vi "Create Rubix Cube in 3D Pic Control.vi"(8 "error in (no error)":errorcluster, 10 "Rubix Array":string[][](array[string])) -> (0 "error out":errorcluster, 2 "Rubix Array":refnum<vi>[][](array[refnum]), 3 "Scene:New Object":refnum<vi>)   [LabVIEW 2019]
uses:
  <vilib>/picture/3D Picture Control/Object/Create Object (name).vi
  <vilib>/picture/3D Picture Control/NI_3D Picture Control.lvlib
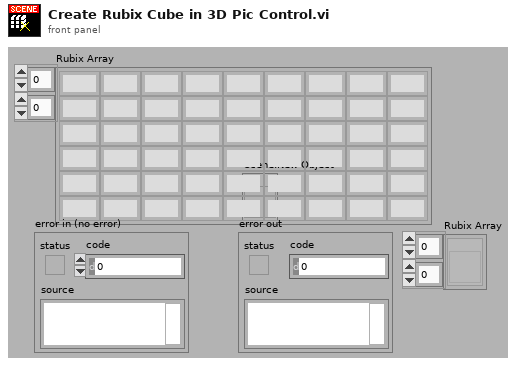
[diagram p1: front panel]
types:
  T1 = cluster{"Axis":cluster{"X":sgl, "Y":sgl, "Z":sgl}, "Angle":sgl}[]
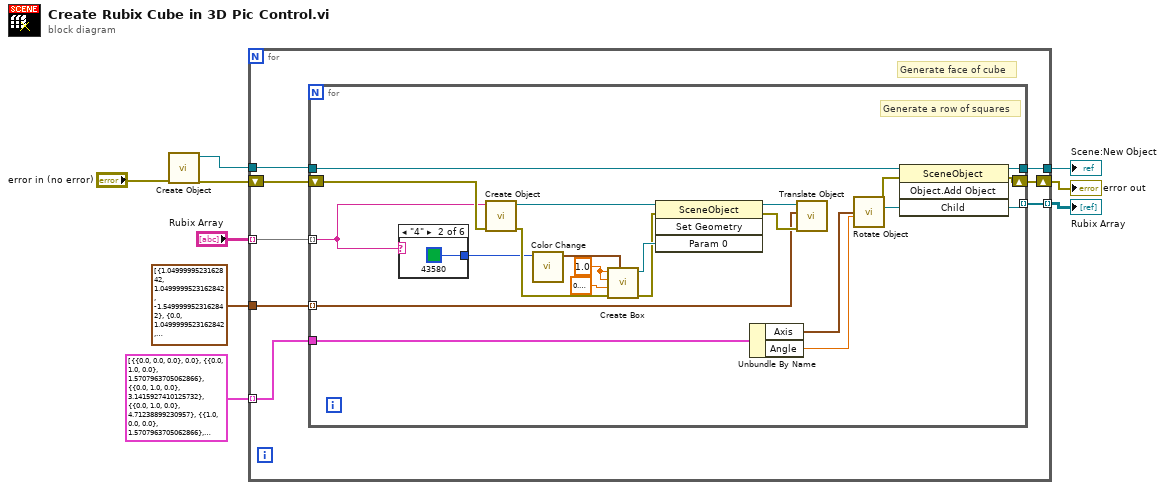
[diagram p0: block diagram]
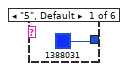
[diagram p2: hidden frame]
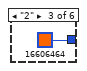
[diagram p3: hidden frame]
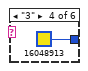
[diagram p4: hidden frame]
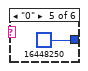
[diagram p5: hidden frame]
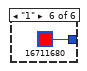
[diagram p6: hidden frame]
diagram:
  n1 = call-poly <vilib>:"Create Object.vi"("error in (no error)"="error in (no error)") -> ("error out"=w6:errorcluster, "Scene:New Object"=w5:refnum<vi>)  [unwired: 9 in]
  n2 = for {
    tunnel: [w17] -> w9
    tunnel: "Rubix Array" -> [w10] mode=indexing
    tunnel: T1 [{"Axis"={"X"=0.0, "Y"=0.0, "Z"=0.0}, "Angle"=0.0}, {"Axis"={"X"=0.0, "Y"=1.0, "Z"=0.0}, "Angle"=1.5707964}, {"Axis"={"X"=0.0, "Y"=1.0, "Z"=0.0}, "Angle"=3.1415927}, {"Axis"={"X"=0.0, "Y"=1.0, "Z"=0.0}, "Angle"=4.712389}, {"Axis"={"X"=1.0, "Y"=0.0, "Z"=0.0}, "Angle"=1.5707964}, {"Axis"={"X"=1.0, "Y"=0.0, "Z"=0.0}, "Angle"=4.712389}] -> [w16] mode=indexing
    tunnel: w5 -> [w15]
    shift-right: [w14] -> w3
    shift-left: w6 -> [w13]
    tunnel: cluster{"X":sgl, "Y":sgl, "Z":sgl}[] [{"X"=1.05, "Y"=1.05, "Z"=-1.55}, {"X"=0.0, "Y"=1.05, "Z"=-1.55}, {"X"=-1.05, "Y"=1.05, "Z"=-1.55}, {"X"=1.05, "Y"=0.0, "Z"=-1.55}, {"X"=0.0, "Y"=0.0, "Z"=-1.55}, {"X"=-1.05, "Y"=0.0, "Z"=-1.55}, {"X"=1.05, "Y"=-1.05, "Z"=-1.55}, {"X"=0.0, "Y"=-1.05, "Z"=-1.55}, {"X"=-1.05, "Y"=-1.05, "Z"=-1.55}] -> [w12]
    tunnel: [w11] -> w1 mode=indexing
    # "Generate face of cube"
    n3 = for {
      tunnel: w12 -> [w26] mode=indexing
      shift-right: [w30] -> w14
      shift-left: w13 -> [w25]
      tunnel: w15 -> [w34]
      tunnel: [w35] -> w17
      tunnel: w10 -> [w22] mode=indexing
      tunnel: w16 -> [w29]
      tunnel: [w23] -> w11 mode=indexing
      w27 = sgl 1.0 ("Length X")
      # "Generate a row of squares"
      n4 = case shown="\"4\"" w22 {
        tunnel: [u32 1388031 ("Color") u32 43580 ("Color") u32 16606464 ("Color") u32 16048913 ("Color") u32 16448250 ("Color") u32 16711680 ("Color")] -> w24
        frame "5", Default {
        }
        frame "4" {
        }
        frame "2" {
        }
        frame "3" {
        }
        frame "0" {
        }
        frame "1" {
        }
      }
      n5 = call-poly <vilib>:"Create Object.vi"("error in (no error)"=w25, "Name"=w22) -> ("error out"=w33:errorcluster, "Scene:New Object"=w38:refnum<vi>)  [unwired: 8 in]
      n6 = call <vilib>:"Color Change.vi"("Color"=w24) -> ("RGBA"=w39:cluster{"R":sgl, "G":sgl, "B":sgl, "A":sgl})  [unwired: 10 in]
      n7 = call <vilib>:"Create Box.vi"("Color"=w39, "error in (no error)"=w33, "Length Z"=sgl 0.1, "Length Y"=w27, "Length X"=w27) -> ("error out"=w32:errorcluster, "New Box Refnum"=w37:refnum<vi>)  [unwired: 5 in]
      n8 = invoke class="SceneObject" method="Set Geometry"(reference=w38, error in=w32, "Param 0"=w37) -> (reference out=w36:refnum<vi>, error out=w31:errorcluster)  [unwired: 1 in, 2 out]
      n9 = Unbundle By Name(w29) -> ("Axis"=w20:cluster{"X":sgl, "Y":sgl, "Z":sgl}, "Angle"=w19:sgl)
      n10 = call <vilib>:"Translate Object.vi"("error in (no error)"=w31, "Translation"=w26, "Scene.Object In"=w36) -> ()  [unwired: 7 in, 2 out]
      n11 = call <vilib>:"Rotate Object.vi"("Angle"=w19, "Axis"=w20) -> ("error out"=w21:errorcluster, "Scene.Object Out"=w18:refnum<vi>)  [unwired: 8 in]
      n12 = invoke class="SceneObject" method="Object.Add Object"(reference=w34, error in=w21, "Child"=w18) -> (reference out=w35:refnum<vi>, error out=w30:errorcluster, "Child"=w23:refnum<vi>)  [unwired: 1 in, 1 out]
    }
  }
  "Scene:New Object" <- w9
  "error out" <- w3
  "Rubix Array" <- w1
